vi "Finish.vi"   [LabVIEW 2018]
doc: "This VI is called just before exiting. It is expected to close I/O refnum, save collected data, etc."
uses:
  <vilib>/Rock Robotics/WPI/Utilities/WPI_GetSetVariantRefNum.vi
types:
  T1 = typedef "WPI_JoystickDevRef.ctl" = cluster{"Device":T2}
  T2 = typedef "WPI_JoystickDeviceEnum.ctl" = enum16{"USB 0", "USB 1", "USB 2", "USB 3", "USB 4", "USB 5"}
  T3 = typedef "WPI_CompressorDevRef.ctl" = cluster{"DevStatus":errorcluster, "Pneumatics Control Module":u8}
  T4 = typedef "WPI_SolenoidDevRef.ctl" = cluster{"DevStatus":errorcluster, "Pneumatics Control Module":u8, "Forward Solenoid Channel":T5, "Reverse Solenoid Channel":T5}
  T5 = typedef "WPI_SolenoidChannel.ctl" = enum8{"Solenoid 0", "Solenoid 1", "Solenoid 2", "Solenoid 3", "Solenoid 4", "Solenoid 5", "Solenoid 6", "Solenoid 7", "Invalid"}
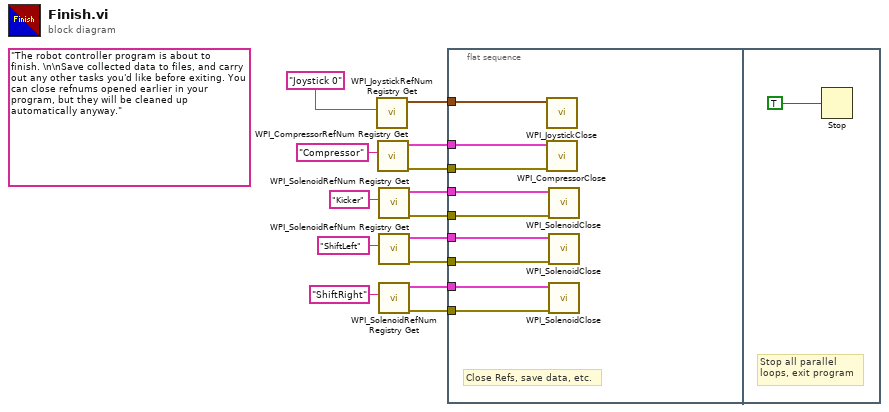
[diagram p0: block diagram]
diagram:
  (unwired) "The robot controller program is about to finish. \n\nSave collected data to files, and carry out any other tasks you'd like before exiting. You can close refnums opened earlier in your program, but they will be cleaned up automatically anyway."
  n1 = call <vilib>:"WPI_JoystickRefNum Registry Get.vi"("refnum name"="Joystick 0") -> ("JoystickDevRef"=w13:T1)  [unwired: 1 in, 9 out]
  n2 = call <vilib>:"WPI_CompressorRefNum Registry Get.vi"("refnum name"="Compressor") -> ("error out"=w11:errorcluster, "CompressorDevRef"=w12:T3)  [unwired: 9 in]
  n3 = call <vilib>:"WPI_SolenoidRefNum Registry Get.vi"("refnum name"="Kicker") -> ("error out"=w9:errorcluster, "SolenoidDevRef"=w8:T4)  [unwired: 9 in]
  n4 = call <vilib>:"WPI_SolenoidRefNum Registry Get.vi"("refnum name"="ShiftLeft") -> ("error out"=w4:errorcluster, "SolenoidDevRef"=w5:T4)  [unwired: 9 in]
  n5 = call <vilib>:"WPI_SolenoidRefNum Registry Get.vi"("refnum name"="ShiftRight") -> ("error out"=w3:errorcluster, "SolenoidDevRef"=w2:T4)  [unwired: 9 in]
  n6 = flat-sequence {
    tunnel: w13 -> [w23]
    tunnel: w12 -> [w22]
    tunnel: w11 -> [w21]
    tunnel: w9 -> [w20]
    tunnel: w8 -> [w19]
    tunnel: w4 -> [w17]
    tunnel: w5 -> [w18]
    tunnel: w3 -> [w16]
    tunnel: w2 -> [w15]
    frame #0 {
      # "Close Refs, save data, etc."
      n7 = call <vilib>:"WPI_JoystickClose.vi"("JoystickDevRef"=w23) -> ()  [unwired: 11 out]
      n8 = call <vilib>:"WPI_CompressorClose.vi"("error in (no error)"=w21, "CompressorDevRef"=w22) -> ()  [unwired: 9 in, 1 out]
      n9 = call <vilib>:"WPI_SolenoidClose.vi"("error in (no error)"=w20, "SolenoidDevRef"=w19) -> ()  [unwired: 9 in, 1 out]
      n10 = call <vilib>:"WPI_SolenoidClose.vi"("error in (no error)"=w17, "SolenoidDevRef"=w18) -> ()  [unwired: 9 in, 1 out]
      n11 = call <vilib>:"WPI_SolenoidClose.vi"("error in (no error)"=w16, "SolenoidDevRef"=w15) -> ()  [unwired: 9 in, 1 out]
    }
    frame #1 {
      # "Stop all parallel\nloops, exit program"
      n12 = Stop(stop? (T)=TRUE ("Quit")) -> ()
    }
  }
